vi "Apply Steering Frame Velocity to Wheels.vi"(5 "wheel indexes":i32[](array[numeric]), 6 "constraint error tolerance (1E-12)":dbl=1e-12, 7 "apply data to motors (F)":bool, 8 "error in (no error)":errorcluster, 10 "steering frame velocity":dbl[](array[numeric])=[0.0, 0.0, 0.0], 11 "steering frame in":refnum<class "NI_Robotics_Steering Frame.lvclass">) -> (0 "error out":errorcluster, 1 "calculated wheel states":T1[](array[typedef]), 2 "coerced steering frame velocity":dbl[](array[numeric]), 3 "steering frame out":refnum<class "NI_Robotics_Steering Frame.lvclass">)   [LabVIEW 2017, in "NI_Robotics_Steering Frame.lvclass"]
doc: "Calculates the state of each wheel necessary to satisfy the <B>steering frame velocity</B> or <B>arc velocity</B> at the center of the steering frame. You must manually select the polymorphic instance to use."
uses:
  <vilib>/robotics/Steering/Steering Frame/NI_Robotics_Steering Frame.lvclass
  <vilib>/robotics/Steering/Wheel/Wheel State.ctl
  <vilib>/robotics/Steering/Steering Frame/NI_Robotics_Steering Frame.lvclass/NI_Robotics_Steering Frame.ctl
  <vilib>/robotics/Steering/Wheel/NI_Robotics_Wheel.lvclass/NI_Robotics_Wheel.ctl
  <vilib>/robotics/Utilities/Generate Error.vi
  <vilib>/robotics/Steering/Wheel/Convert Steering Frame Velocity to Wheel Frame.vi
  <vilib>/robotics/Steering/Wheel/Apply Wheel State to Motors.vi
  <vilib>/robotics/Steering/Wheel/Create Wheel Angular Velocity Row_Frame.vi
  <vilib>/robotics/Steering/Wheel/Create Caster Angular Velocity Row_Frame.vi
  <vilib>/Analysis/baseanly.llb/A x Vector.vi
  <vilib>/robotics/Steering/Wheel/NI_Robotics_Wheel.lvclass
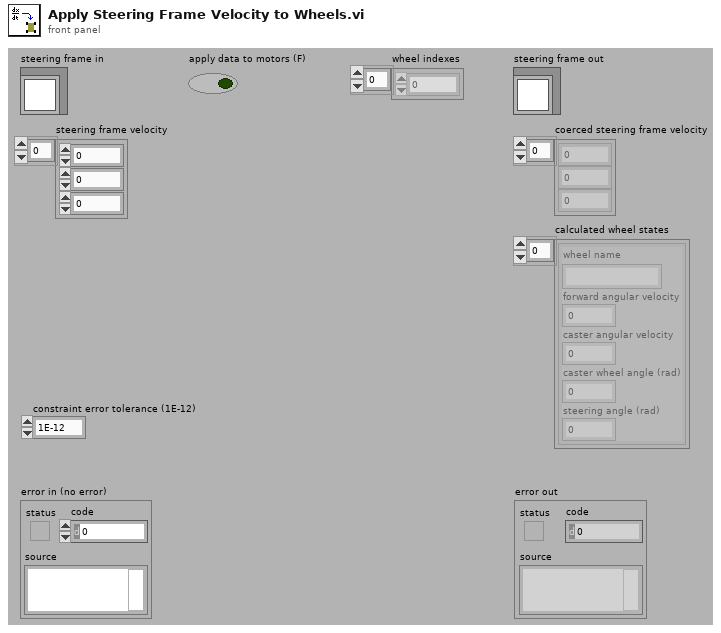
[diagram p1: front panel]
types:
  T1 = typedef "NI_Robotics_Wheel.lvclass/Wheel State.ctl" = cluster{"wheel name":string, "forward angular velocity":dbl, "caster angular velocity":dbl, "caster wheel angle (rad)":dbl, "steering angle (rad)":dbl}
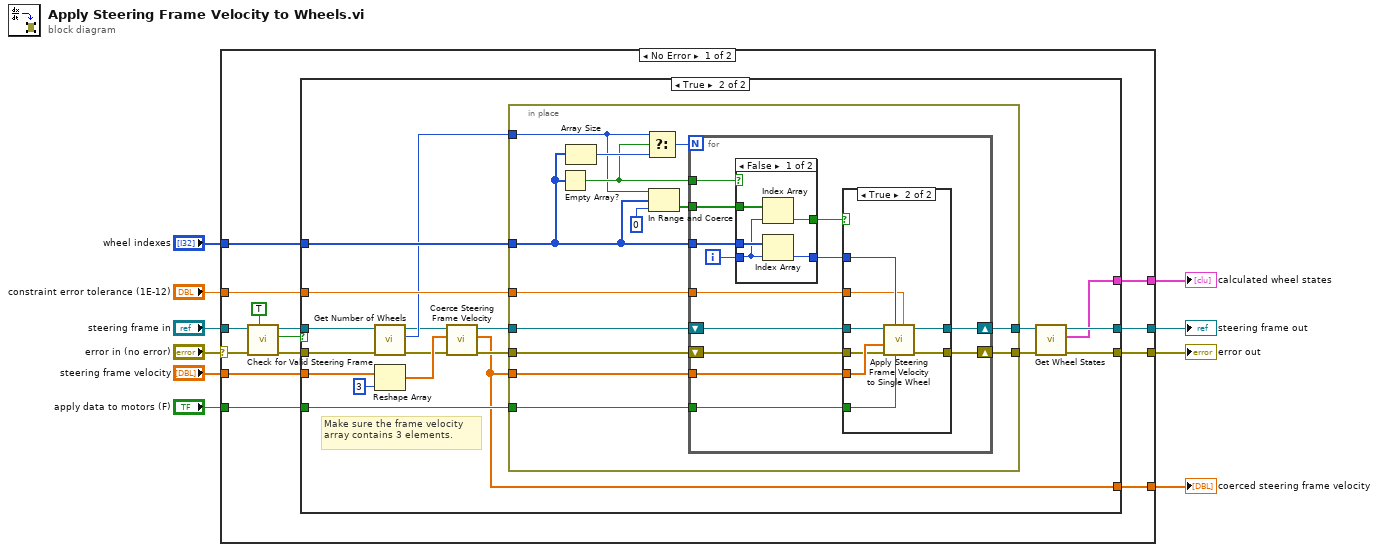
[diagram p0: block diagram]
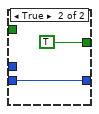
[diagram p4: hidden frame]
diagram:
  n1 = case shown="No Error" "error in (no error)" {
    selector: "error in (no error)" -> [w15 w91]
    tunnel: [w22 w91] -> w9
    tunnel: [w20 w90] -> w7
    tunnel: "steering frame in" -> [w17 w90]
    tunnel: "steering frame velocity" -> [w18 _]
    tunnel: [w19 _] -> w5
    tunnel: "constraint error tolerance (1E-12)" -> [w24 _]
    tunnel: [w23 _] -> w3
    tunnel: "apply data to motors (F)" -> [w21 _]
    tunnel: "wheel indexes" -> [w11 _]
    frame No Error {
      n2 = call <vilib>:"Check for Valid Steering Frame.vi"("produce error if invalid (T)"=TRUE, "error in (no error)"=w15, "steering frame in"=w17) -> ("error out"=w14:errorcluster, "valid?"=w13:bool, "steering frame out"=w16:refnum<class "NI_Robotics_Steering Frame.lvclass">)  [unwired: 6 in]
      n3 = case shown="True" w13 {
        tunnel: w24 -> [_ w45]
        tunnel: [_ w34] -> w23
        tunnel: [w25 w33] -> w22
        tunnel: w21 -> [_ w44]
        tunnel: [w26 w36] -> w20
        tunnel: [_ w39] -> w19
        tunnel: w18 -> [_ w41]
        tunnel: w16 -> [w26 w30]
        tunnel: w14 -> [w25 w28]
        tunnel: w11 -> [_ w38]
        frame False {
        }
        frame True {
          # "Make sure the frame velocity array contains 3 elements."
          n4 = call <vilib>:"Get Number of Wheels.vi"("error in (no error)"=w28, "steering frame in"=w30) -> ("error out"=w27:errorcluster, "number of wheels"=w31:i32, "steering frame out"=w29:refnum<class "NI_Robotics_Steering Frame.lvclass">)  [unwired: 7 in]
          n5 = Reshape Array(w41, 3 ("dimension size")) -> (w40:dbl[])
          n6 = call-dynamic "Coerce Steering Frame Velocity.vi"("error in (no error)"=w27, "steering frame velocity"=w40, "steering frame in"=w29) -> ("error out"=w43:errorcluster, "coerced steering frame velocity"=w39:dbl[], "steering frame out"=w37:refnum<class "NI_Robotics_Steering Frame.lvclass">)  [unwired: 6 in]
          n7 = in-place {
            in-place-border: w45 -> [w59]
            in-place-border: w43 -> [w58]
            in-place-border: [w57] -> w32
            in-place-border: w44 -> [w55]
            in-place-border: w39 -> [w56]
            in-place-border: w38 -> [w51]
            in-place-border: w31 -> [w48]
            in-place-border: w37 -> [w47]
            in-place-border: [w46] -> w35
            n8 = Empty Array?(array=w51) -> (empty?=w52:bool)
            n9 = Array Size(array=w51) -> (size(s)=w53:i32)
            n10 = Select(t=w48, s=w52, f=w53) -> (s? t:f=w54:i32)
            n11 = In Range and Coerce(upper limit=w48, x=w51, lower limit=0) -> (In Range?=w49:bool[])  [unwired: 1 out]
            n12 = for {
              N: w54 -> [_]
              tunnel: w59 -> [w72]
              tunnel: w56 -> [w71]
              shift-right: [w69] -> w57
              shift-left: w58 -> [w70]
              tunnel: w55 -> [w68]
              tunnel: w51 -> [w66]
              tunnel: w52 -> [w67]
              tunnel: w49 -> [w63]
              shift-right: [w60] -> w46
              shift-left: w47 -> [w61]
              i -> [w65]
              n13 = case shown="False" w67 {
                tunnel: w66 -> [w87 _]
                tunnel: w65 -> [w85 w89]
                tunnel: [w84 w89] -> w64
                tunnel: w63 -> [w86 _]
                tunnel: [w83 TRUE ("lower limit")] -> w62
                frame False {
                  n14 = Index Array(array=w86, index=w85) -> (element=w83:bool)
                  n15 = Index Array(array=w87, index=w85) -> (element=w84:i32)
                }
                frame True {
                }
              }
              n16 = case shown="True" w62 {
                tunnel: w72 -> [_ w79]
                tunnel: w71 -> [_ w81]
                tunnel: w70 -> [w74 w78]
                tunnel: [w74 w77] -> w69
                tunnel: w68 -> [_ w80]
                tunnel: w64 -> [_ w82]
                tunnel: w61 -> [w73 w76]
                tunnel: [w73 w75] -> w60
                frame False {
                }
                frame True {
                  n17 = call <vilib>:"Apply Steering Frame Velocity to Single Wheel.vi"("constraint error tolerance (1E-12)"=w79, "apply data to motors"=w80, "wheel index"=w82, "error in (no error)"=w78, "steering frame velocity"=w81, "steering frame in"=w76) -> ("error out"=w77:errorcluster, "steering frame out"=w75:refnum<class "NI_Robotics_Steering Frame.lvclass">)  [unwired: 4 in]
                }
              }
            }
          }
          n18 = call <vilib>:"Get Wheel States.vi"("error in (no error)"=w32, "steering frame in"=w35) -> ("error out"=w33:errorcluster, "wheel states"=w34:T1[], "steering frame out"=w36:refnum<class "NI_Robotics_Steering Frame.lvclass">)  [unwired: 7 in]
        }
      }
    }
    frame Error {
    }
  }
  "error out" <- w9
  "steering frame out" <- w7
  "coerced steering frame velocity" <- w5
  "calculated wheel states" <- w3
